vi "Decode Message.vi"(8 "Error In":errorcluster, 11 "Image 2 Path in":path) -> (0 "Error Out":errorcluster, 3 "Decoded Message":string)   [LabVIEW 2020]
doc: "Decodes the encoded image, extracting the LSB of the image red, blue, and green components. Looks for the sequence \"###\" to know when to stop decoding."
uses:
  Image Comparison/Image Comparison.lvclass
panel:
  out "Numeric":i32
  out "size(s)":i32
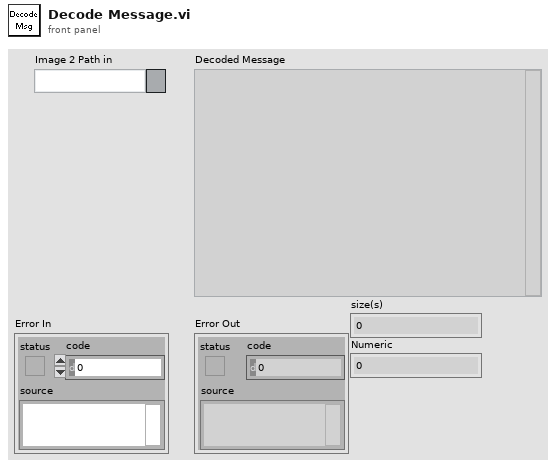
[diagram p1: front panel]
types:
  T1 = typedef "imagedata.ctl" = cluster{"image type":i32, "image depth":i32, "image":u8[], "mask":u8[], "colors":u32[], "Rectangle":cluster{"left":i16, "top":i16, "right":i16, "bottom":i16}}
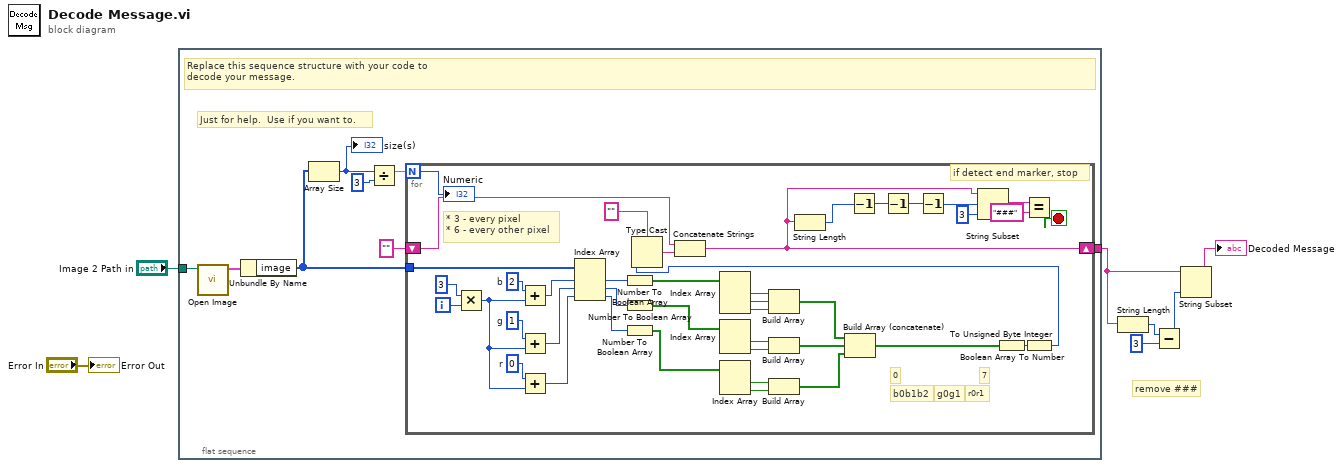
[diagram p0: block diagram]
diagram:
  # "remove ###"
  n1 = flat-sequence {
    tunnel: [w8] -> w5
    tunnel: "Image 2 Path in" -> [w15]
    frame #0 {
      # "Just for help.  Use if you want to."
      # "Replace this sequence structure with your code to \ndecode your message."
      n2 = call "Open Image.vi"("Image"=w15) -> ("image data"=w14:T1)  [unwired: 9 in, 1 out]
      n3 = Unbundle By Name(w14) -> ("image"=w10:u8[])
      n4 = Array Size(array=w10) -> (size(s)=w13:i32)
      "size(s)" <- w13
      n5 = Divide(x=w13, y=3) -> (x/y=w11:dbl)
      n6 = for {
        N: w11 -> [w50]
        tunnel: w10 -> [w54]
        shift-right: [w19] -> w8
        shift-left: "" -> [w52]
        i -> [w57]
        stop <- w16 stop-if-true
        w47 = 0  # r
        w48 = 1  # g
        w55 = 2  # b
        # "7"
        # "0"
        # "if detect end marker, stop"
        # "g0g1"
        # "r0r1"
        # "b0b1b2"
        # "* 3 - every pixel\n* 6 - every other pixel"
        n7 = Multiply(x=3, y=w57) -> (x*y=w44:i32)
        n8 = Add(x=w55, y=w44) -> (x+y=w49:i32)
        n9 = Add(x=w48, y=w44) -> (x+y=w46:i32)
        n10 = Add(x=w47, y=w44) -> (x+y=w45:i32)
        n11 = Index Array(array=w54, index #1=w49, index #2=w46, index #3=w45) -> (element #1=w43:u8, element #2=w42:u8, element #3=w41:u8)
        n12 = Number To Boolean Array(number=w43) -> (Boolean array=w40:bool[])
        n13 = Number To Boolean Array(number=w42) -> (Boolean array=w39:bool[])
        n14 = Number To Boolean Array(number=w41) -> (Boolean array=w38:bool[])
        n15 = Index Array(array=w40) -> (element #1=w37:bool, element #2=w36:bool, element #3=w35:bool)  [unwired: 3 in]
        n16 = Index Array(array=w39) -> (element #1=w34:bool, element #2=w33:bool)  [unwired: 2 in]
        n17 = Index Array(array=w38) -> (element #1=w32:bool, element #2=w31:bool)  [unwired: 2 in]
        n18 = Build Array(w37, w36, w35) -> (w26:bool[])
        n19 = Build Array(w34, w33) -> (w30:bool[])
        n20 = Build Array(w32, w31) -> (w25:bool[])
        n21 = Build Array (concatenate)(w26, w30, w25) -> (w29:bool[])
        n22 = Boolean Array To Number(Boolean array=w29) -> (number=w28:u32)
        n23 = To Unsigned Byte Integer(number=w28) -> (unsigned 8bit integer=w27:u8)
        n24 = Type Cast(type="", x=w27) -> (*(type *) &x=w51:string)
        n25 = Concatenate Strings(w52, w51) -> (w19:string)
        n26 = String Length(string=w19) -> (length=w24:i32)
        n27 = Decrement(x=w24) -> (x-1=w23:i32)
        n28 = Decrement(x=w23) -> (x-1=w22:i32)
        n29 = Decrement(x=w22) -> (x-1=w21:i32)
        n30 = String Subset(string=w19, offset (0)=w21, length (rest)=3 ("length (rest)")) -> (substring=w18:string)
        n31 = Equal?(x=w18, y="###") -> (x = y?=w16:bool)
        "Numeric" <- w50
      }
    }
  }
  n32 = String Length(string=w5) -> (length=w4:i32)
  n33 = Subtract(x=w4, y=3) -> (x-y=w2:i32)
  n34 = String Subset(string=w5, length (rest)=w2) -> (substring=→"Decoded Message":string)  [unwired: 1 in]
  "Error Out" <- "Error In"
